vi "Close.vi"(8 "error in (no error)":errorcluster, 11 "Reply Protocol Base in":refnum<class "Reply Protocol Base.lvclass">) -> (0 "error out":errorcluster, 3 "Reply Protocol Base out":refnum<class "Reply Protocol Base.lvclass">)   [LabVIEW 2023, in "HAL GOOP4.lvlib" / "Reply Protocol Base.lvclass"]
uses:
  Reply Protocol Base.lvclass
  Reply Protocol Base.lvclass/Reply Protocol Base.ctl
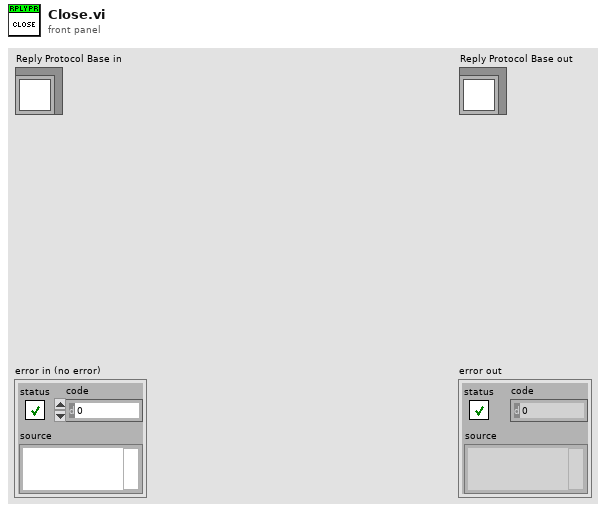
[diagram p1: front panel]
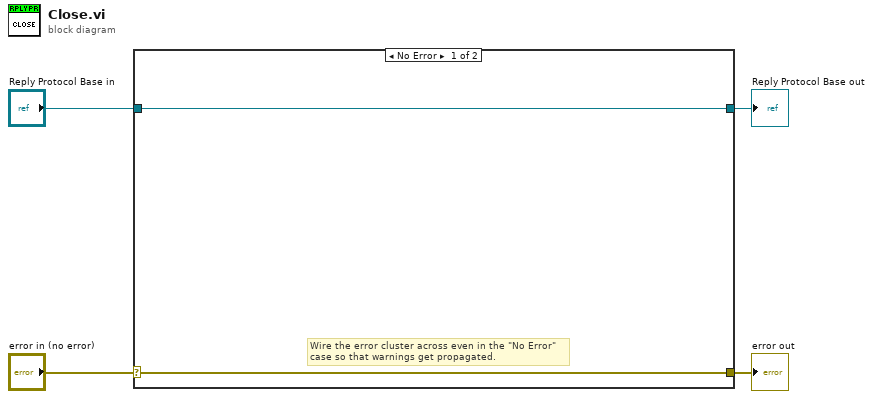
[diagram p0: block diagram]
diagram:
  n1 = case shown="No Error" "error in (no error)" {
    selector: "error in (no error)" -> [w5 w8]
    tunnel: [w5 w8] -> w3
    tunnel: [w6 w7] -> w1
    tunnel: "Reply Protocol Base in" -> [w6 w7]
    frame No Error {
      # "Wire the error cluster across even in the \"No Error\"\ncase so that warnings get propagated."
    }
    frame Error {
    }
  }
  "error out" <- w3
  "Reply Protocol Base out" <- w1
